vi "DeferActorCorePanel.vi"(8 "error in (no error)":errorcluster, 10 "On/Off":bool, 11 "CameraTestingUI in":refnum<class "CameraTestingUI.lvclass">) -> (0 "error out":errorcluster, 3 "CameraTestingUI out":refnum<class "CameraTestingUI.lvclass">)   [LabVIEW 2020, in "CameraTestingUI.lvlib" / "CameraTestingUI.lvclass"]
uses:
  CameraTestingUI.lvclass
  CameraTestingUI.lvclass/CameraTestingUI.ctl
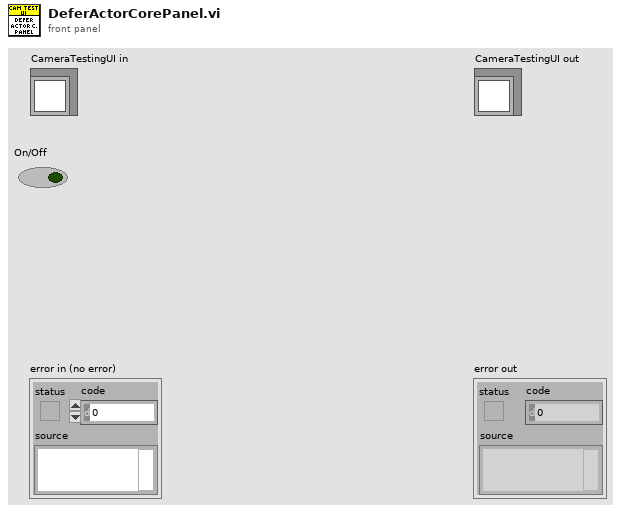
[diagram p1: front panel]
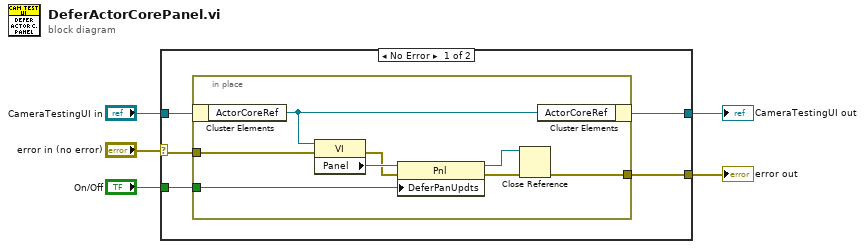
[diagram p0: block diagram]
diagram:
  n1 = case shown="No Error" "error in (no error)" {
    selector: "error in (no error)" -> [w7 w20]
    tunnel: [w10 w20] -> w1
    tunnel: "CameraTestingUI in" -> [w9 w19]
    tunnel: [w8 w19] -> w3
    tunnel: "On/Off" -> [w6 _]
    frame No Error {
      n2 = in-place {
        in-place-border: [w13] -> w10
        in-place-border: w7 -> [w12]
        in-place-border: w6 -> [w11]
        n3 = in-place-cluster #1(w9) -> ("ActorCoreRef"=w17:refnum<vi>)
        n4 = property class="VI"(reference=w17, error in=w12) -> (error out=w16:errorcluster, "Panel"=w18:refnum<vi>)  [unwired: 1 out]
        n5 = property class="Pnl"(reference=w18, error in=w16, "DeferPanUpdts"=w11) -> (reference out=w14:refnum<vi>, error out=w15:errorcluster)
        n6 = Close Reference(reference=w14, error in (no error)=w15) -> (error out=w13:errorcluster)
        n7 = in-place-cluster #1("ActorCoreRef"=w17) -> (w8:refnum<class "CameraTestingUI.lvclass">)
      }
    }
    frame Error {
    }
  }
  "error out" <- w1
  "CameraTestingUI out" <- w3
